vi "Switch Interface.vi"() -> ()   [LabVIEW 2011]
uses:
  SubVI/Pumps_Valves_Dependencies_Global.vi
panel:
  in  "Mode of Operation":bool
  out "Towing tank Volume":dbl
  out "Salt Saturator":dbl(slide) scale=0.0..100.0
  out "B":dbl(slide) scale=0.0..100.0
  out "A":dbl(slide) scale=0.0..100.0
  out "Density Meter":dbl
  out "D":dbl(slide) scale=0.0..100.0
  out "C":dbl(slide) scale=0.0..100.0
  in  "?":bool
  in  "Valve Power":bool
  in  "Pump Power":bool
  in  "Main Rack Power":bool
  in  "V34":bool
  in  "V32":bool
  in  "V19":bool
  in  "V33":bool
  in  "V18":bool
  in  "V20":bool
  in  "V26":bool
  in  "V25":bool
  in  "V24":bool
  in  "V23":bool
  in  "V22":bool
  in  "V21":bool
  in  "V27":bool
  in  "V28":bool
  in  "V31":bool
  in  "V13":bool
  in  "V15":bool
  in  "V11":bool
  in  "V10":bool
  in  "V9":bool
  in  "V14":bool
  in  "V8":bool
  in  "V6":bool
  in  "V7":bool
  in  "V12":bool
  in  "V5":bool
  in  "V4":bool
  in  "V30":bool
  in  "V29":bool
  in  "Pump D":bool
  in  "Pump C":bool
  in  "Pump B":bool
  in  "Pump A":bool
  out "Fresh Water":dbl(slide) scale=0.0..10.0
  out "Brine":dbl(slide) scale=0.0..10.0
  # "DRAIN"
  # "DRAIN"
  # "WATER SUPPLY"
  # "DRAIN"
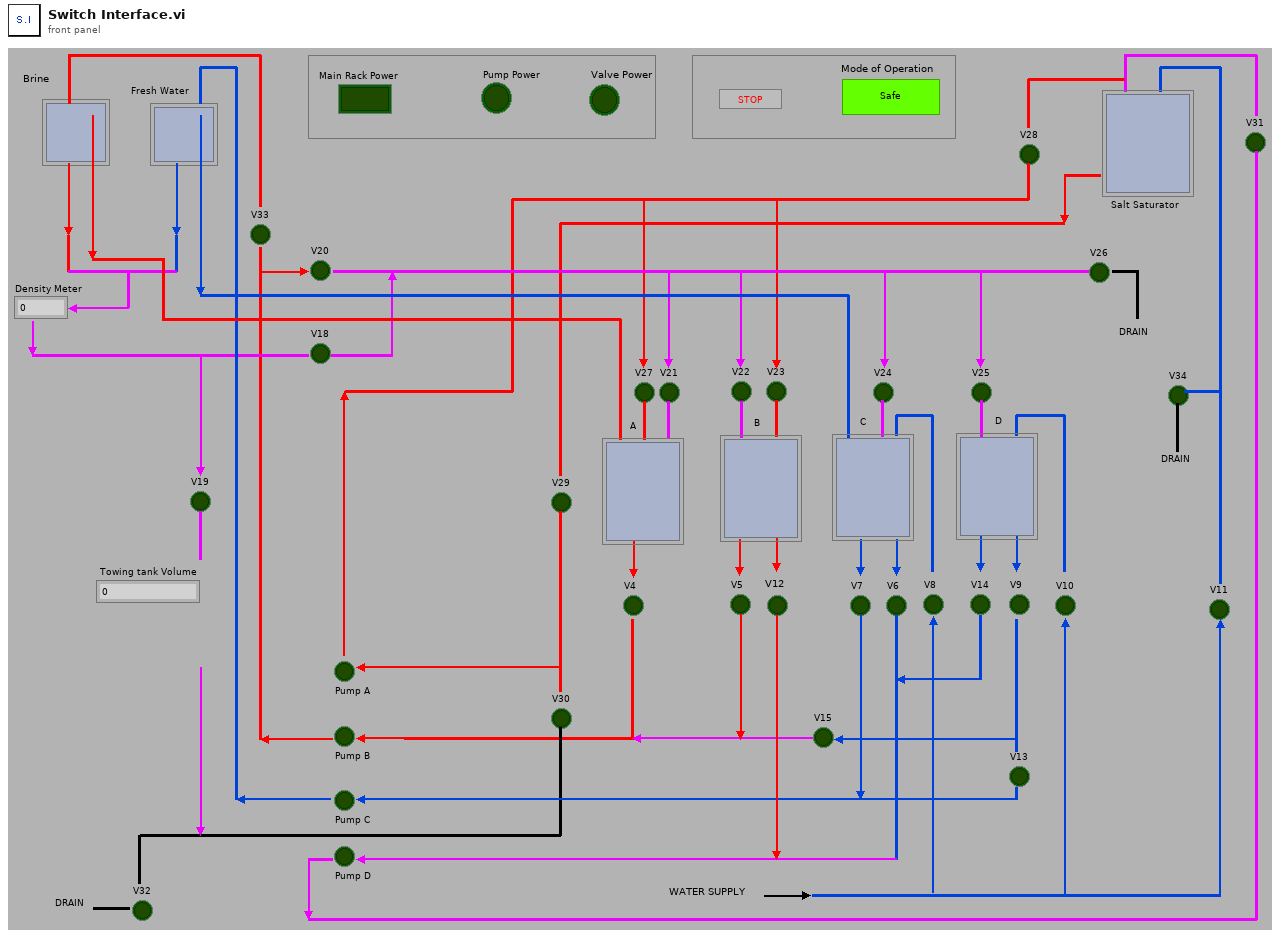
[diagram p1: front panel]
types:
  T1 = typedef "Valve_Pump.ctl" = enum16{"Main Rack Power", "Pump Power", "Valve Power", "V4", "V5", "V6", "V7", "V8", "V9", "V10", "V11", "V12", "V13", "V14", "V15", "V18", "V19", "V20", "V21", "V22", "V23", "V24", "V25", "V26", "V27", "V28", "V29", "V30", "V31", "V32", "V33", "V34", "Pump A", "Pump B", "Pump C", "Pump D"}
  T2 = cluster{"Height Array[0]":dbl, "Height Array[1]":dbl, "Height Array[2]":dbl, "Height Array[3]":dbl, "Height Array[4]":dbl}
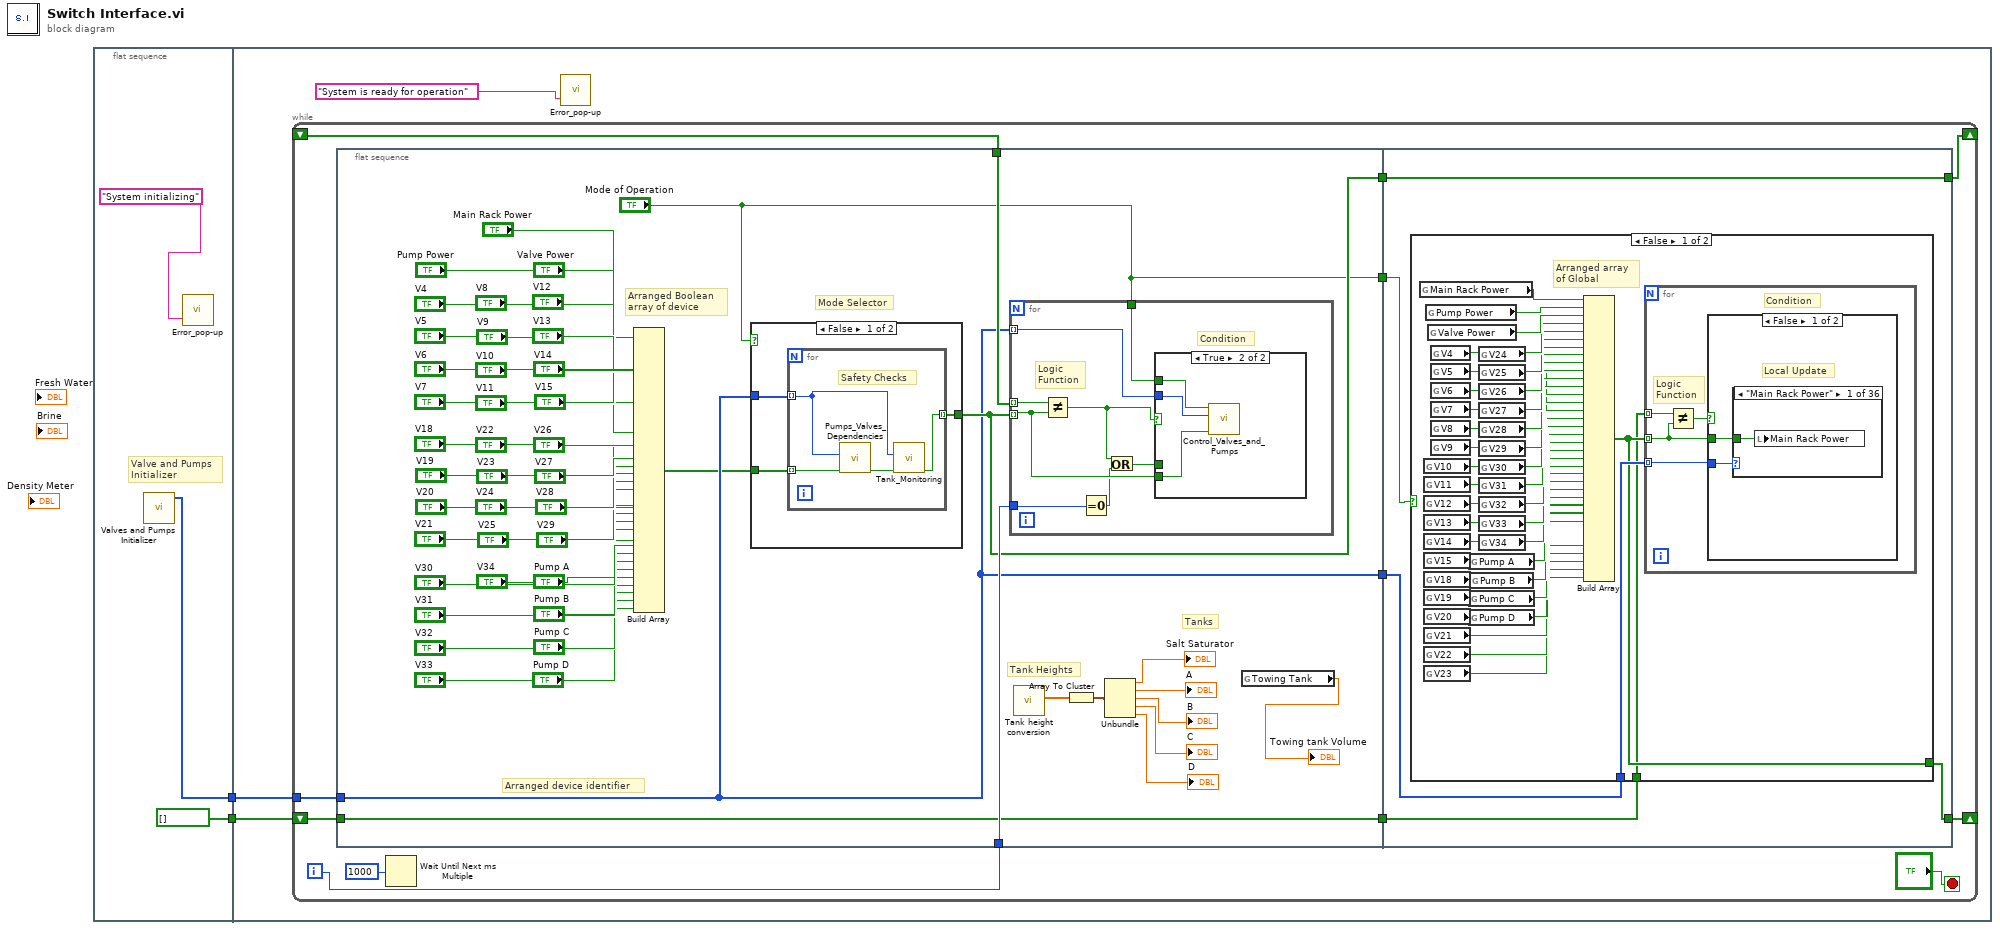
[diagram p0: block diagram]
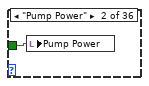
[diagram p4: hidden frame]
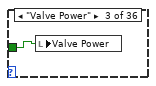
[diagram p5: hidden frame]
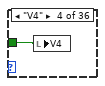
[diagram p6: hidden frame]
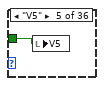
[diagram p7: hidden frame]
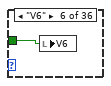
[diagram p8: hidden frame]
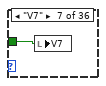
[diagram p9: hidden frame]
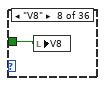
[diagram p10: hidden frame]
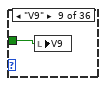
[diagram p11: hidden frame]
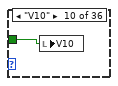
[diagram p12: hidden frame]
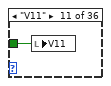
[diagram p13: hidden frame]
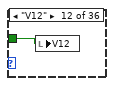
[diagram p14: hidden frame]
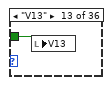
[diagram p15: hidden frame]
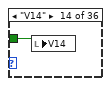
[diagram p16: hidden frame]
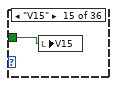
[diagram p17: hidden frame]
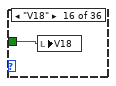
[diagram p18: hidden frame]
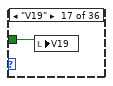
[diagram p19: hidden frame]
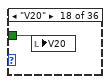
[diagram p20: hidden frame]
diagram:
  n1 = flat-sequence {
    tunnel: [w4] -> w2
    tunnel: [bool[] []] -> w1
    tunnel: w2 -> [w8]
    tunnel: w1 -> [w7]
    frame #0 {
      # "Valve and Pumps\nInitializer"
      n2 = call "Valves and Pumps Initializer.vi"() -> ("Devices"=w4:T1[])  [unwired: 11 in]
      n3 = call "Error_pop-up.vi"("New msg"="System initializing") -> ()  [unwired: 2 in]
    }
    frame #1 {
      n4 = while {
        shift-right: [w13] -> _
        shift-left: _ -> [w19]
        tunnel: w8 -> [w12]
        shift-right: [w11] -> _
        shift-left: w7 -> [w9]
        i -> [w18]
        stop <- "?" stop-if-true
        n5 = flat-sequence {
          tunnel: w19 -> [w71]
          tunnel: w18 -> [w70]
          tunnel: [w54] -> w16
          tunnel: [w53] -> w15
          tunnel: ["Mode of Operation"] -> w14
          tunnel: w12 -> [w53]
          tunnel: [w52] -> w10
          tunnel: w9 -> [w52]
          tunnel: [w95] -> w13
          tunnel: w16 -> [w95]
          tunnel: w15 -> [w94]
          tunnel: w14 -> [w93]
          tunnel: [w92] -> w11
          tunnel: w10 -> [w91]
          frame #0 {
            # "Tanks"
            # "Arranged device identifier"
            # "Tank Heights"
            # "Arranged Boolean \narray of device"
            # "Mode Selector"
            n6 = Build Array("Main Rack Power", "Pump Power", "Valve Power", "V4", "V5", "V6", "V7", "V8", "V9", "V10", "V11", "V12", "V13", "V14", "V15", "V18", "V19", "V20", "V21", "V22", "V23", "V24", "V25", "V26", "V27", "V28", "V29", "V30", "V31", "V32", "V33", "V34", "Pump A", "Pump B", "Pump C", "Pump D") -> (w22:bool[])
            n7 = case shown="False" "Mode of Operation" {
              tunnel: w22 -> [w74 w79]
              tunnel: [w73 w79] -> w54
              tunnel: w53 -> [w72 _]
              frame False {
                n8 = for {
                  tunnel: w74 -> [w78] mode=indexing
                  tunnel: [w75] -> w73 mode=indexing
                  tunnel: w72 -> [w77] mode=indexing
                  # "Safety Checks"
                  n9 = call "Pumps_Valves_Dependencies.vi"("Set state:"=w78, "Device"=w77) -> ("State"=w76:bool)  [unwired: 9 in]
                  n10 = call "Tank_Monitoring.vi"("Set state:"=w76, "Device"=w77) -> ("Set"=w75:bool)  [unwired: 9 in]
                }
              }
              frame True {
              }
            }
            n11 = for {
              tunnel: w53 -> [w85] mode=indexing
              tunnel: w54 -> [w84] mode=indexing
              tunnel: w71 -> [w83] mode=indexing
              tunnel: w70 -> [w81]
              tunnel: "Mode of Operation" -> [w80]
              # "Logic\nFunction"
              # "Condition"
              n12 = Not Equal?(x=w83, y=w84) -> (x != y?=w87:bool)
              n13 = Equal To 0?(x=w81) -> (x = 0?=w82:bool)
              n14 = Or(x=w87, y=w82) -> (x .or. y?=w86:bool)
              n15 = case shown="True" w87 {
                tunnel: w85 -> [_ w90]
                tunnel: w86 -> [_ _]
                tunnel: w84 -> [_ w89]
                tunnel: w80 -> [_ w88]
                frame False {
                }
                frame True {
                  n16 = call "Control_Valves_and_Pumps.vi"("Set state:"=w89, "Device"=w90, "Mode of Operation"=w88) -> ()  [unwired: 9 in]
                }
              }
            }
            n17 = call "Tank height conversion.vi"() -> ("Height Array"=w45:dbl[])  [unwired: 11 in]
            n18 = Array To Cluster(array=w45) -> (cluster=w51:T2)
            n19 = Unbundle(w51) -> ("Height Array[0]"=→"Salt Saturator":dbl, "Height Array[1]"=→"A":dbl, "Height Array[2]"=→"B":dbl, "Height Array[3]"=→"C":dbl, "Height Array[4]"=→"D":dbl)
            n20 = global read "Pumps_Valves_Dependencies_Global.vi" "Towing Tank"() -> (→"Towing tank Volume":dbl)
          }
          frame #1 {
            n21 = case shown="False" w93 {
              tunnel: w94 -> [w134 _]
              tunnel: [w97 w177] -> w92
              tunnel: w91 -> [w96 w177]
              frame False {
                # "Arranged array\nof Global"
                n22 = global read "Pumps_Valves_Dependencies_Global.vi" "Main Rack Power"() -> (w133:bool)
                n23 = global read "Pumps_Valves_Dependencies_Global.vi" "V10"() -> (w124:bool)
                n24 = global read "Pumps_Valves_Dependencies_Global.vi" "V11"() -> (w123:bool)
                n25 = global read "Pumps_Valves_Dependencies_Global.vi" "V12"() -> (w122:bool)
                n26 = global read "Pumps_Valves_Dependencies_Global.vi" "V13"() -> (w121:bool)
                n27 = global read "Pumps_Valves_Dependencies_Global.vi" "V14"() -> (w120:bool)
                n28 = global read "Pumps_Valves_Dependencies_Global.vi" "V15"() -> (w119:bool)
                n29 = global read "Pumps_Valves_Dependencies_Global.vi" "V18"() -> (w118:bool)
                n30 = global read "Pumps_Valves_Dependencies_Global.vi" "V19"() -> (w117:bool)
                n31 = global read "Pumps_Valves_Dependencies_Global.vi" "V20"() -> (w116:bool)
                n32 = global read "Pumps_Valves_Dependencies_Global.vi" "V21"() -> (w115:bool)
                n33 = global read "Pumps_Valves_Dependencies_Global.vi" "V22"() -> (w114:bool)
                n34 = global read "Pumps_Valves_Dependencies_Global.vi" "V23"() -> (w113:bool)
                n35 = global read "Pumps_Valves_Dependencies_Global.vi" "Pump Power"() -> (w132:bool)
                n36 = global read "Pumps_Valves_Dependencies_Global.vi" "Valve Power"() -> (w131:bool)
                n37 = global read "Pumps_Valves_Dependencies_Global.vi" "V4"() -> (w130:bool)
                n38 = global read "Pumps_Valves_Dependencies_Global.vi" "V5"() -> (w129:bool)
                n39 = global read "Pumps_Valves_Dependencies_Global.vi" "V6"() -> (w128:bool)
                n40 = global read "Pumps_Valves_Dependencies_Global.vi" "V7"() -> (w127:bool)
                n41 = global read "Pumps_Valves_Dependencies_Global.vi" "V8"() -> (w126:bool)
                n42 = global read "Pumps_Valves_Dependencies_Global.vi" "V9"() -> (w125:bool)
                n43 = global read "Pumps_Valves_Dependencies_Global.vi" "Pump A"() -> (w101:bool)
                n44 = global read "Pumps_Valves_Dependencies_Global.vi" "Pump C"() -> (w99:bool)
                n45 = global read "Pumps_Valves_Dependencies_Global.vi" "Pump D"() -> (w98:bool)
                n46 = global read "Pumps_Valves_Dependencies_Global.vi" "Pump B"() -> (w100:bool)
                n47 = global read "Pumps_Valves_Dependencies_Global.vi" "V24"() -> (w112:bool)
                n48 = global read "Pumps_Valves_Dependencies_Global.vi" "V25"() -> (w111:bool)
                n49 = global read "Pumps_Valves_Dependencies_Global.vi" "V26"() -> (w110:bool)
                n50 = global read "Pumps_Valves_Dependencies_Global.vi" "V27"() -> (w109:bool)
                n51 = global read "Pumps_Valves_Dependencies_Global.vi" "V28"() -> (w108:bool)
                n52 = global read "Pumps_Valves_Dependencies_Global.vi" "V29"() -> (w107:bool)
                n53 = global read "Pumps_Valves_Dependencies_Global.vi" "V30"() -> (w106:bool)
                n54 = global read "Pumps_Valves_Dependencies_Global.vi" "V31"() -> (w105:bool)
                n55 = global read "Pumps_Valves_Dependencies_Global.vi" "V32"() -> (w104:bool)
                n56 = global read "Pumps_Valves_Dependencies_Global.vi" "V33"() -> (w103:bool)
                n57 = global read "Pumps_Valves_Dependencies_Global.vi" "V34"() -> (w102:bool)
                n58 = Build Array(w133, w132, w131, w130, w129, w128, w127, w126, w125, w124, w123, w122, w121, w120, w119, w118, w117, w116, w115, w114, w113, w112, w111, w110, w109, w108, w107, w106, w105, w104, w103, w102, w101, w100, w99, w98) -> (w97:bool[])
                n59 = for {
                  tunnel: w97 -> [w136] mode=indexing
                  tunnel: w134 -> [w137] mode=indexing
                  tunnel: w96 -> [w135] mode=indexing
                  # "Logic\nFunction"
                  # "Condition"
                  n60 = Not Equal?(x=w135, y=w136) -> (x != y?=w138:bool)
                  n61 = case shown="False" w138 {
                    tunnel: w137 -> [w140 _]
                    tunnel: w136 -> [w139 _]
                    frame False {
                      # "Local Update"
                      n62 = case shown="\"Main Rack Power\"" w140 {
                        tunnel: w139 -> [w141 w142 w143 w144 w145 w146 w147 w148 w149 w150 w151 w152 w153 w154 w155 w156 w157 w158 w159 w160 w161 w162 w163 w164 w165 w166 w167 w168 w169 w170 w171 w172 w173 w174 w175 w176]
                        frame "Main Rack Power" {
                          n63 = local write "Main Rack Power"(w141) -> ()
                        }
                        frame "Pump Power" {
                          n64 = local write "Pump Power"(w142) -> ()
                        }
                        frame "Valve Power" {
                          n65 = local write "Valve Power"(w143) -> ()
                        }
                        frame "V4" {
                          n66 = local write "V4"(w144) -> ()
                        }
                        frame "V5" {
                          n67 = local write "V5"(w145) -> ()
                        }
                        frame "V6" {
                          n68 = local write "V6"(w146) -> ()
                        }
                        frame "V7" {
                          n69 = local write "V7"(w147) -> ()
                        }
                        frame "V8" {
                          n70 = local write "V8"(w148) -> ()
                        }
                        frame "V9" {
                          n71 = local write "V9"(w149) -> ()
                        }
                        frame "V10" {
                          n72 = local write "V10"(w150) -> ()
                        }
                        frame "V11" {
                          n73 = local write "V11"(w151) -> ()
                        }
                        frame "V12" {
                          n74 = local write "V12"(w152) -> ()
                        }
                        frame "V13" {
                          n75 = local write "V13"(w153) -> ()
                        }
                        frame "V14" {
                          n76 = local write "V14"(w154) -> ()
                        }
                        frame "V15" {
                          n77 = local write "V15"(w155) -> ()
                        }
                        frame "V18" {
                          n78 = local write "V18"(w156) -> ()
                        }
                        frame "V19" {
                          n79 = local write "V19"(w157) -> ()
                        }
                        frame "V20" {
                          n80 = local write "V20"(w158) -> ()
                        }
                        frame "V21" {
                          n81 = local write "V21"(w159) -> ()
                        }
                        frame "V22" {
                          n82 = local write "V22"(w160) -> ()
                        }
                        frame "V23" {
                          n83 = local write "V23"(w161) -> ()
                        }
                        frame "V24" {
                          n84 = local write "V24"(w162) -> ()
                        }
                        frame "V25" {
                          n85 = local write "V25"(w163) -> ()
                        }
                        frame "V26" {
                          n86 = local write "V26"(w164) -> ()
                        }
                        frame "V27" {
                          n87 = local write "V27"(w165) -> ()
                        }
                        frame "V28" {
                          n88 = local write "V28"(w166) -> ()
                        }
                        frame "V29" {
                          n89 = local write "V29"(w167) -> ()
                        }
                        frame "V30" {
                          n90 = local write "V30"(w168) -> ()
                        }
                        frame "V31" {
                          n91 = local write "V31"(w169) -> ()
                        }
                        frame "V32" {
                          n92 = local write "V32"(w170) -> ()
                        }
                        frame "V33" {
                          n93 = local write "V33"(w171) -> ()
                        }
                        frame "V34" {
                          n94 = local write "V34"(w172) -> ()
                        }
                        frame "Pump A" {
                          n95 = local write "Pump A"(w173) -> ()
                        }
                        frame "Pump B" {
                          n96 = local write "Pump B"(w174) -> ()
                        }
                        frame "Pump C" {
                          n97 = local write "Pump C"(w175) -> ()
                        }
                        frame "Pump D" {
                          n98 = local write "Pump D"(w176) -> ()
                        }
                      }
                    }
                    frame True {
                    }
                  }
                }
              }
              frame True {
              }
            }
          }
        }
        n99 = Wait Until Next ms Multiple(millisecond multiple=u32 1000) -> ()  [unwired: 1 out]
      }
      n100 = call "Error_pop-up.vi"("New msg"="System is ready for operation") -> ()  [unwired: 2 in]
    }
  }
